vi "SGUI Set Multiple UIntegers By Label.vi"(6 "error in":errorcluster, 8 "labels (empty)":string, 9 "format (empty)":string, 10 "integers (empty)":u32[](array[numeric])) -> (7 "error out":errorcluster, 11 "control references out":refnum<vi>[](array[refnum]))   [LabVIEW 2020, in "varilib.lvlib"]
doc: "This VI sets value(s) and format(s) of numeric controls designated by label(s) name string. Multiple can be assigned at once by using multiline string 'labels'. One line per control. If empty format string is entered, format stays unchanged. If empty values array is entered, no value is modified. If multiple controls are assigned but just one number or format string is assigned, the same format or/and value is written to all controls.\nNote: NaN numeric value is ignored - it is used as no modify value!\n\nThi VI ignores input errors (will execute anyway) however will generate error if any of the named controls is not found or writting to it fails (invalid type of control)."
uses:
  varilib.lvlib
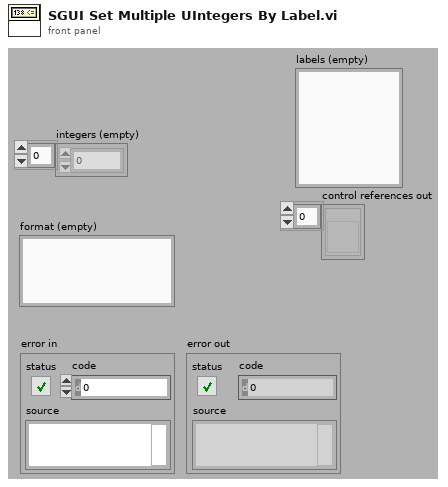
[diagram p1: front panel]
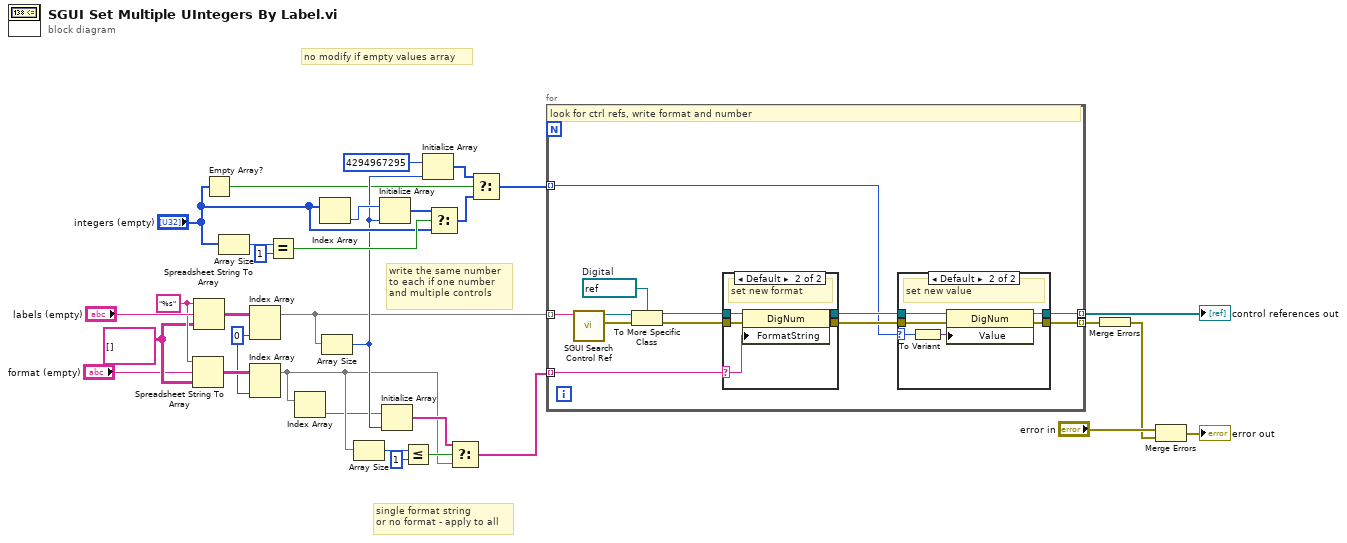
[diagram p0: block diagram]
diagram:
  w3 = 0 ("disabled index (col)")
  w25 = string[][] []
  w26 = "%s"
  # "write the same number\nto each if one number\nand multiple controls"
  # "no modify if empty values array"
  # "single format string\nor no format - apply to all"
  n1 = Spreadsheet String To Array(format string=w26, spreadsheet string="format (empty)", array type (2D Dbl)=w25) -> (array=w22:string[][])  [unwired: 1 in]
  n2 = Spreadsheet String To Array(format string=w26, spreadsheet string="labels (empty)", array type (2D Dbl)=w25) -> (array=w20:string[][])  [unwired: 1 in]
  n3 = Empty Array?(array="integers (empty)") -> (empty?=w5:bool)
  n4 = Array Size(array="integers (empty)") -> (size(s)=w14:i32)
  n5 = Index Array(array=w20, index (col)=w3) -> (element=w4:string[])  [unwired: 1 in]
  n6 = Index Array(array=w22, index (col)=w3) -> (element=w2:string[])  [unwired: 1 in]
  n7 = Equal?(x=w14, y=1) -> (x = y?=w11:bool)
  n8 = Index Array(array=w2) -> (element=w1:string)  [unwired: 1 in]
  n9 = Index Array(array="integers (empty)") -> (element=w9:u32)  [unwired: 1 in]
  n10 = Array Size(array=w4) -> (size(s)=w6:i32)
  n11 = Array Size(array=w2) -> (size(s)=w24:i32)
  n12 = Initialize Array(w9, w6) -> (w10:u32[])
  n13 = Initialize Array(w1, w6) -> (w19:string[])
  n14 = Less Or Equal?(x=w24, y=1) -> (x <= y?=w17:bool)
  n15 = Initialize Array(u32 4294967295, w6) -> (w16:u32[])
  n16 = Select(t=w10, s=w11, f="integers (empty)") -> (s? t:f=w12:u32[])
  n17 = Select(t=w19, s=w17, f=w2) -> (s? t:f=w18:string[])
  n18 = Select(t=w16, s=w5, f=w12) -> (s? t:f=w7:u32[])
  n19 = for {
    tunnel: w4 -> [w44] mode=indexing
    tunnel: [w39] -> w31 mode=indexing
    tunnel: [w40] -> w32 mode=indexing
    tunnel: w18 -> [w43] mode=indexing
    tunnel: w7 -> [w33] mode=indexing
    w36 = refnum<vi> refnum  # Digital
    # "look for ctrl refs, write format and number"
    n20 = call "SGUI Search Control Ref.vi"("control label (empty)"=w44) -> ("error out"=w38:errorcluster, "control ref out"=w37:refnum<vi>)  [unwired: 8 in, 1 out]
    n21 = To More Specific Class(target class=w36, reference=w37, error in=w38) -> (specific class reference=w34:refnum<vi>, error out=w35:errorcluster)
    n22 = case shown="Default" w43 {
      selector: w43 -> [_ w55]
      tunnel: w35 -> [w54 w59]
      tunnel: [w54 w58] -> w42
      tunnel: [w53 w57] -> w41
      tunnel: w34 -> [w53 w56]
      frame "" {
      }
      frame Default {
        # "set new format"
        n23 = property class="DigNum"(reference=w56, error in=w59, "FormatString"=w55) -> (reference out=w57:refnum<vi>, error out=w58:errorcluster)
      }
    }
    n24 = case shown="Default" w33 {
      selector: w33 -> [_ w47]
      tunnel: w42 -> [w46 w52]
      tunnel: [w46 w51] -> w40
      tunnel: [w45 w50] -> w39
      tunnel: w41 -> [w45 w49]
      frame -1 {
      }
      frame Default {
        # "set new value"
        n25 = To Variant(anything=w47) -> (Variant=w48:variant)
        n26 = property class="DigNum"(reference=w49, error in=w52, "Value"=w48) -> (reference out=w50:refnum<vi>, error out=w51:errorcluster)
      }
    }
  }
  "control references out" <- w31
  n27 = Merge Errors(w32) -> (w27:errorcluster)
  n28 = Merge Errors("error in", w27) -> (→"error out":errorcluster)
